vi "Drive Execute.vi"   [LabVIEW 2016]
uses:
  Drive Control Type.ctl
  Drive Notifier.ctl
  <vilib>/Rock Robotics/WPI/DriverStation/WPI_DriverStationRobotMode2.ctl
  Drive Globals.vi
  Robot Global Data.vi
types:
  T1 = typedef "WPI_MotorControlDeviceRef.ctl" = cluster{"DeviceStatus":errorcluster, "Type":T2, "PWM":cluster{"PWM Channel":T3, "DeadBand":T4}, "CAN":cluster{"Device Number":u8, "SetOutput VI Ref":variant, "GetOutput VI Ref":variant, "Enable VI Ref":variant, "Disable VI Ref":variant, "Data":variant}, "Invert":bool}
  T2 = typedef "WPI_MotorControlType.ctl" = enum16{"PWM", "CAN"}
  T3 = typedef "FPGA_DIOPWMChannel.ctl" = enum8{"PWM 0", "PWM 1", "PWM 2", "PWM 3", "PWM 4", "PWM 5", "PWM 6", "PWM 7", "PWM 8", "PWM 9", "PWM MXP 0", "PWM MXP 1", "PWM MXP 2", "PWM MXP 3", "PWM MXP 4", "PWM MXP 5", "PWM MXP 6", "PWM MXP 7", "PWM MXP 8", "PWM MXP 9", "Invalid"}
  T4 = typedef "WPI_PWMDeadband.ctl" = cluster{"Name":string, "maxPositivePwm":i32, "minPositivePwm":i32, "centerPwm":i32, "maxNegativePwm":i32, "minNegativePwm":i32, "angularRange":u16}
  T5 = typedef "Drive Control Type.ctl" = enum16{"No Op", "Fieldcentric", "Robotcentric", "Reset Wheel Position", "Reset Gyro Value", "Turn to Angle", "Drive For Time", "Drive For Time2"}
  T6 = typedef "WPI_DriverStationRobotMode2.ctl" = enum16{"Autonomous Disabled", "Autonomous Enabled", "Teleop Disabled", "Teleop Enabled", "Disconnected", "Finish", "Test Disabled", "Test Enabled", "Emergency Stopped"}
  T7 = typedef "Drive Notifier.ctl" = cluster{"Parameter 1":dbl, "Parameter 2":dbl, "Parameter 3":dbl, "Drive Control List":T5, "Parameter 4":dbl, "Gear Angle":dbl, "Parameter 6":dbl, "Parameter 7":dbl, "Parameter 8":dbl, "Parameter 9":dbl, "Robotcentric":bool, "Reset Gyro":bool, "Reset Wheels":bool, "Turn to Gear Left":bool, "Turn to Gear Center":bool, "Turn to Gear Right":bool, "Half Power":bool, "Drive Notifier":refnum<notifier>, "Step":i32}
  T8 = typedef "WPI_CANTalonSRX_GlobalStatus.ctl" = cluster{"Applied Throttle":dbl, "Module Enabled":bool, "CAN Error":errorcluster, "Closed Loop Error":dbl, "Forward Limit Switch Closed":bool, "Reverse Limit Switch Closed":bool, "Sensor Position":dbl, "Sensor Velocity":dbl, "Current":dbl, "Sticky Fault - Over Temp":bool, "Sticky Fault - Under Voltage":bool, "Sticky Fault - Forward Limit":bool, "Sticky Fault - Reverse Limit":bool, "Sticky Fault - Forward Soft Limit":bool, "Sticky Fault - Reverse Soft Limit":bool, "Brake is Enabled":bool, "Encoder Position":dbl, "Encoder Velocity":dbl, "Encoder Index Count":dbl, "Encoder A Pin State":bool, "Encoder B Pin State":bool, "Encoder Index Pin State":bool, "Analog In":dbl, "Analog In Velocity":dbl, "Temperature (C)":dbl, "Battery Voltage":dbl, "Control 5 Is Supported":bool, "Current Profile Slot Select":dbl, "Pos Div 8":bool, "Vel Div 4":bool, "Pulse Width Position":i32, "Pulse Width Velocity":i32, "Pulse Width Rise To Rise (us)":i32, "Pulse Width Rise To Fall (us)":i32, "Mot Prof Active Is Under Run":bool, "Mot Prof Active Has Under Run":bool, "Mot Prof Active Is Last":bool, "Mot Prof Active Velocity Only":bool, "Mot Prof Active Is Valid":bool, "Mot Prof Buffer Is Full":bool, "Mot Prof Active Profile Slot Select":i32, "Mot Prof NextID":i32, "Mot Prof Count":i32, "Mot Prof Active Velocity":dbl, "Mot Prof Active Position":dbl, "Mot Prof Output Enable":i32, "UsageFrame":u32, "Motion Magic Active Trajectory":cluster{"Velocity":dbl, "Position":dbl}}
  T9 = typedef "CTRE_PigeonIMU_DeviceRef.ctl" = cluster{"DeviceStatus":errorcluster, "Device Number":u8, "Type":T10, "Device ID":u32}
  T10 = typedef "CTRE_PigeonIMU_ConnectionType.ctl" = u32
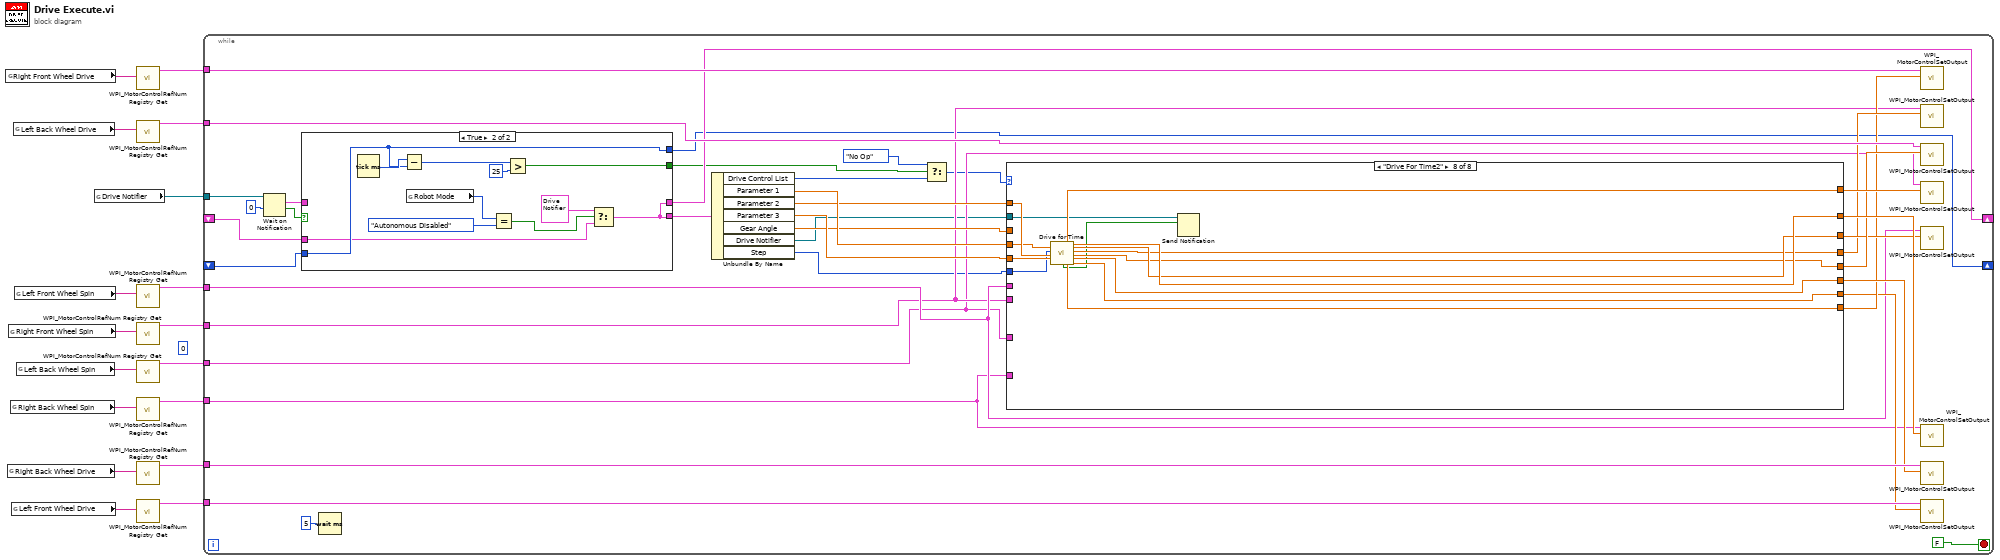
[diagram p0: block diagram]
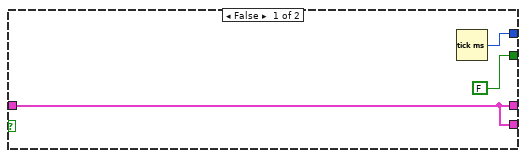
[diagram p2: hidden frame]
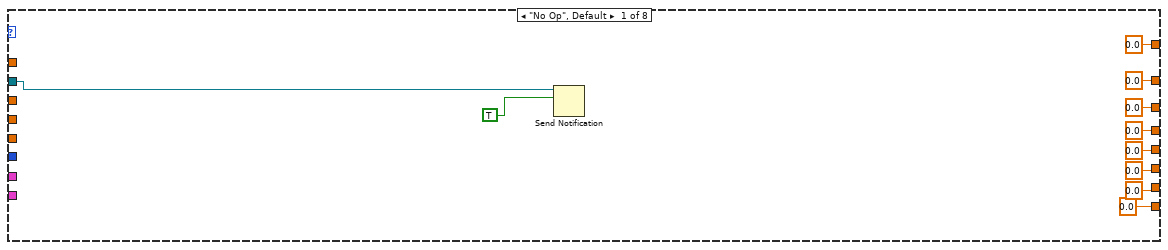
[diagram p3: hidden frame]
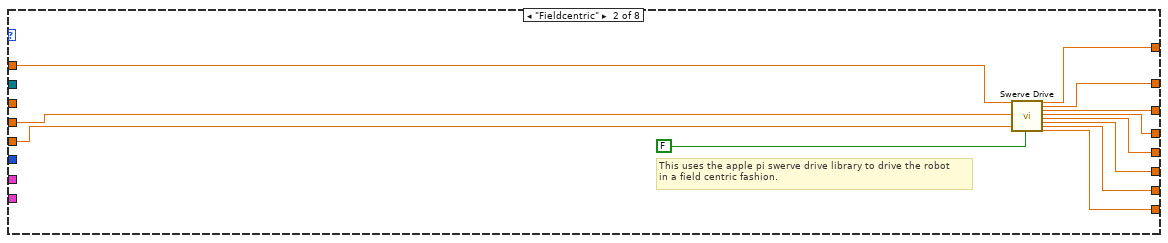
[diagram p4: hidden frame]
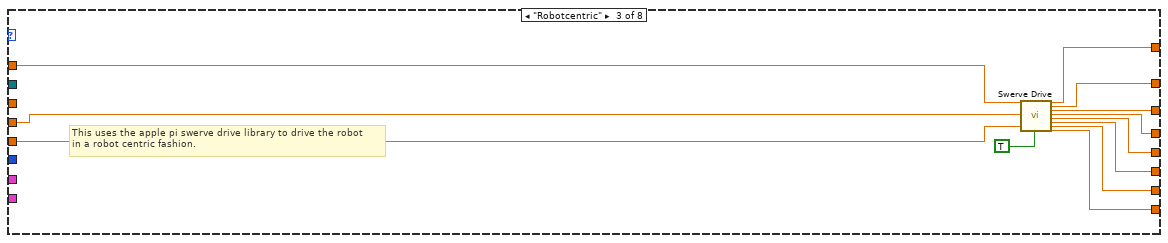
[diagram p5: hidden frame]
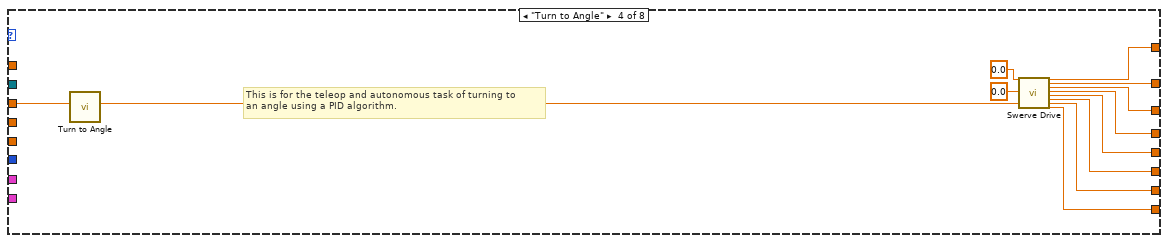
[diagram p6: hidden frame]
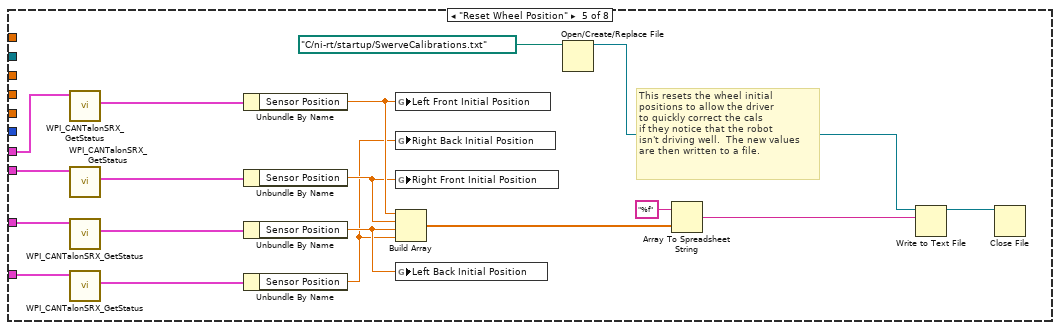
[diagram p7: hidden frame]
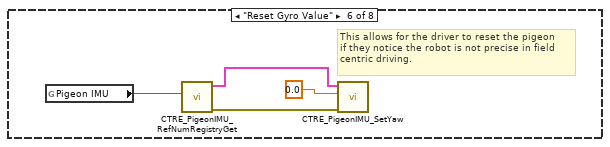
[diagram p8: hidden frame]
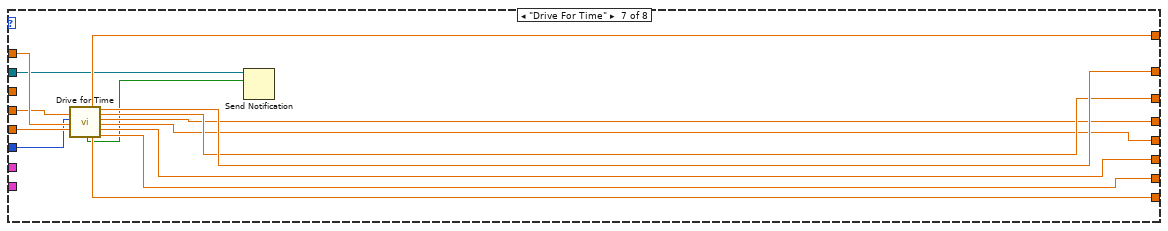
[diagram p9: hidden frame]
diagram:
  (unwired) 0
  n1 = global read "Drive Globals.vi" "Right Front Wheel Drive"() -> (w12:string)
  n2 = global read "Drive Globals.vi" "Right Back Wheel Drive"() -> (w11:string)
  n3 = global read "Drive Globals.vi" "Right Front Wheel Spin"() -> (w8:string)
  n4 = global read "Drive Globals.vi" "Right Back Wheel Spin"() -> (w6:string)
  n5 = global read "Drive Globals.vi" "Left Front Wheel Drive"() -> (w13:string)
  n6 = global read "Drive Globals.vi" "Left Back Wheel Drive"() -> (w10:string)
  n7 = global read "Drive Globals.vi" "Left Front Wheel Spin"() -> (w9:string)
  n8 = global read "Drive Globals.vi" "Left Back Wheel Spin"() -> (w7:string)
  n9 = global read "Drive Globals.vi" "Drive Notifier"() -> (w17:refnum<notifier>)
  n10 = call <vilib>:"WPI_MotorControlRefNum Registry Get.vi"("refnum name"=w12) -> ("MotorControlDevRef"=w2:T1)  [unwired: 9 in, 1 out]
  n11 = call <vilib>:"WPI_MotorControlRefNum Registry Get.vi"("refnum name"=w10) -> ("MotorControlDevRef"=w15:T1)  [unwired: 9 in, 1 out]
  n12 = call <vilib>:"WPI_MotorControlRefNum Registry Get.vi"("refnum name"=w9) -> ("MotorControlDevRef"=w1:T1)  [unwired: 9 in, 1 out]
  n13 = call <vilib>:"WPI_MotorControlRefNum Registry Get.vi"("refnum name"=w8) -> ("MotorControlDevRef"=w3:T1)  [unwired: 9 in, 1 out]
  n14 = call <vilib>:"WPI_MotorControlRefNum Registry Get.vi"("refnum name"=w7) -> ("MotorControlDevRef"=w4:T1)  [unwired: 9 in, 1 out]
  n15 = call <vilib>:"WPI_MotorControlRefNum Registry Get.vi"("refnum name"=w6) -> ("MotorControlDevRef"=w5:T1)  [unwired: 9 in, 1 out]
  n16 = call <vilib>:"WPI_MotorControlRefNum Registry Get.vi"("refnum name"=w11) -> ("MotorControlDevRef"=w14:T1)  [unwired: 9 in, 1 out]
  n17 = call <vilib>:"WPI_MotorControlRefNum Registry Get.vi"("refnum name"=w13) -> ("MotorControlDevRef"=w16:T1)  [unwired: 9 in, 1 out]
  n18 = while {
    tunnel: w17 -> [w49]
    tunnel: w16 -> [w46]
    tunnel: w15 -> [w44]
    tunnel: w14 -> [w45]
    tunnel: w5 -> [w32]
    tunnel: w4 -> [w33]
    tunnel: w3 -> [w34]
    tunnel: w2 -> [w47]
    tunnel: w1 -> [w35]
    shift-right: [w27] -> _
    shift-left: _ -> [w26]
    shift-right: [w25] -> _
    shift-left: _ -> [w24]
    stop <- FALSE stop-if-true
    n19 = Wait on Notification(notifier=w49, timeout in ms (-1)=0) -> (notification=w29:T7, timed out?=w19:bool)  [unwired: 2 in, 2 out]
    n20 = case shown="True" w19 {
      tunnel: w29 -> [w57 _]
      tunnel: [w57 w58] -> w28
      tunnel: [w57 w58] -> w27
      tunnel: w26 -> [_ w59]
      tunnel: [w56 w67] -> w25
      tunnel: w24 -> [_ w67]
      tunnel: [FALSE w64] -> w23
      frame False {
        n21 = Tick Count (ms)() -> (millisecond timer value=w56:u32)
      }
      frame True {
        n22 = Tick Count (ms)() -> (millisecond timer value=w68:u32)
        n23 = Subtract(x=w68, y=w67) -> (x-y=w66:u32)
        n24 = global read "Robot Global Data.vi" "Robot Mode"() -> (w63:T6)
        n25 = Equal?(x=w63, y=WPI_DriverStationRobotMode2."Autonomous Disabled") -> (x = y?=w61:bool)
        n26 = Greater?(x=w66, y=u32 25) -> (0:w64:bool)
        n27 = Select(t=T7 {"Parameter 1"=0.0, "Parameter 2"=0.0, "Parameter 3"=0.0, "Drive Control List"=enum."No Op", "Parameter 4"=0.0, "Gear Angle"=0.0, "Parameter 6"=0.0, "Parameter 7"=0.0, "Parameter 8"=0.0, "Parameter 9"=0.0, "Robotcentric"=FALSE, "Reset Gyro"=FALSE, "Reset Wheels"=FALSE, "Turn to Gear Left"=FALSE, "Turn to Gear Center"=FALSE, "Turn to Gear Right"=FALSE, "Half Power"=FALSE, "Drive Notifier"=refnum, "Step"=0} ("Drive Notifier"), s=w61, f=w59) -> (s? t:f=w58:T7)
      }
    }
    n28 = Wait (ms)(milliseconds to wait=u32 5) -> ()  [unwired: 1 out]
    n29 = Unbundle By Name(w28) -> ("Drive Control List"=w20:T5, "Parameter 1"=w52:dbl, "Parameter 2"=w51:dbl, "Parameter 3"=w50:dbl, "Gear Angle"=w48:dbl, "Drive Notifier"=w31:refnum<notifier>, "Step"=w18:i32)
    n30 = Select(t=Drive_Control_Type."No Op" ("f"), s=w23, f=w20) -> (s? t:f=w22:T5)
    n31 = case shown="\"Drive For Time2\"" w22 {
      tunnel: w52 -> [_ w89 w101 _ _ _ w149 w163]
      tunnel: w51 -> [_ w90 w102 _ _ _ w150 w164]
      tunnel: w50 -> [_ w88 w100 _ _ _ w148 w162]
      tunnel: w48 -> [_ _ _ w113 _ _ _ _]
      tunnel: [0.0 ("Back Left Spin Power") w87 w99 w105 _ _ w147 w161] -> w43
      tunnel: [0.0 ("Back Right Spin Power") w86 w98 w109 _ _ w146 w160] -> w42
      tunnel: [0.0 ("Back Left Motor Power") w85 w97 w108 _ _ w143 w157] -> w41
      tunnel: [0.0 ("Back Right Motor Power") w84 w96 w110 _ _ w142 w156] -> w40
      tunnel: [0.0 ("Front Left Spin Power") w83 w95 w104 _ _ w145 w159] -> w39
      tunnel: [0.0 ("Front Right Spin Power") w82 w94 w106 _ _ w144 w158] -> w38
      tunnel: [0.0 ("Front Right Motor Power") w81 w93 w107 _ _ w140 w154] -> w37
      tunnel: [0.0 ("Front Left Motor Power") w80 w92 w103 _ _ w141 w155] -> w36
      tunnel: w35 -> [_ _ _ _ w118 _ _ _]
      tunnel: w34 -> [_ _ _ _ w117 _ _ _]
      tunnel: w33 -> [_ _ _ _ w116 _ _ _]
      tunnel: w32 -> [_ _ _ _ w115 _ _ _]
      tunnel: w31 -> [w70 _ _ _ _ _ w139 w153]
      tunnel: w18 -> [_ _ _ _ _ _ w137 w151]
      frame "No Op", Default {
        n32 = Send Notification(notification=TRUE, notifier=w70) -> ()  [unwired: 1 in, 2 out]
      }
      frame "Fieldcentric" {
        # "This uses the apple pi swerve drive library to drive the robot\nin a field centric fashion."
        n33 = call "Swerve Drive.vi"("X"=w90, "Y"=w89, "Z"=w88, "Robot-Centric"=FALSE) -> ("Back Left Spin Power"=w87:dbl, "Back Right Spin Power"=w86:dbl, "Front Left Spin Power"=w83:dbl, "Front Right Spin Power"=w82:dbl, "Back Left Motor Power"=w85:dbl, "Back Right Motor Power"=w84:dbl, "Front Left Motor Power"=w80:dbl, "Front Right Motor Power"=w81:dbl)  [unwired: 16 in]
      }
      frame "Robotcentric" {
        # "This uses the apple pi swerve drive library to drive the robot\nin a robot centric fashion."
        n34 = call "Swerve Drive.vi"("X"=w102, "Y"=w101, "Z"=w100, "Robot-Centric"=TRUE) -> ("Back Left Spin Power"=w99:dbl, "Back Right Spin Power"=w98:dbl, "Front Left Spin Power"=w95:dbl, "Front Right Spin Power"=w94:dbl, "Back Left Motor Power"=w97:dbl, "Back Right Motor Power"=w96:dbl, "Front Left Motor Power"=w92:dbl, "Front Right Motor Power"=w93:dbl)  [unwired: 16 in]
      }
      frame "Turn to Angle" {
        # "This is for the teleop and autonomous task of turning to \nan angle using a PID algorithm."
        n35 = call "Turn to Angle.vi"("Target Angle"=w113) -> ("Output Rotation"=w114:dbl)  [unwired: 10 in]
        n36 = call "Swerve Drive.vi"("X"=0.0, "Y"=0.0, "Z"=w114) -> ("Back Left Spin Power"=w105:dbl, "Back Right Spin Power"=w109:dbl, "Front Left Spin Power"=w104:dbl, "Front Right Spin Power"=w106:dbl, "Back Left Motor Power"=w108:dbl, "Back Right Motor Power"=w110:dbl, "Front Left Motor Power"=w103:dbl, "Front Right Motor Power"=w107:dbl)  [unwired: 17 in]
      }
      frame "Reset Wheel Position" {
        # "This resets the wheel initial\npositions to allow the driver\nto quickly correct the cals\nif they notice that the robot\nisn't driving well.  The new values \nare then written to a file."
        n37 = call <vilib>:"WPI_CANTalonSRX_GetStatus.vi"("CAN Talon SRX Ref"=w118) -> ("Talon SRX Status"=w130:T8)  [unwired: 8 in, 2 out]
        n38 = call <vilib>:"WPI_CANTalonSRX_GetStatus.vi"("CAN Talon SRX Ref"=w117) -> ("Talon SRX Status"=w131:T8)  [unwired: 8 in, 2 out]
        n39 = call <vilib>:"WPI_CANTalonSRX_GetStatus.vi"("CAN Talon SRX Ref"=w116) -> ("Talon SRX Status"=w132:T8)  [unwired: 8 in, 2 out]
        n40 = call <vilib>:"WPI_CANTalonSRX_GetStatus.vi"("CAN Talon SRX Ref"=w115) -> ("Talon SRX Status"=w129:T8)  [unwired: 8 in, 2 out]
        n41 = Unbundle By Name(w130) -> ("Sensor Position"=w128:dbl)
        n42 = Unbundle By Name(w131) -> ("Sensor Position"=w127:dbl)
        n43 = Unbundle By Name(w132) -> ("Sensor Position"=w126:dbl)
        n44 = Unbundle By Name(w129) -> ("Sensor Position"=w125:dbl)
        n45 = global write "Drive Globals.vi" "Left Front Initial Position"(w128) -> ()
        n46 = global write "Drive Globals.vi" "Right Back Initial Position"(w125) -> ()
        n47 = global write "Drive Globals.vi" "Right Front Initial Position"(w127) -> ()
        n48 = Build Array(w128, w127, w126, w125) -> (w124:dbl[])
        n49 = global write "Drive Globals.vi" "Left Back Initial Position"(w126) -> ()
        n50 = Open/Create/Replace File(file path (use dialog)=path "C:/ni-rt/startup/SwerveCalibrations.txt" ("file (use dialog)")) -> (refnum out=w121:refnum<file>)  [unwired: 5 in, 2 out]
        n51 = Array To Spreadsheet String(array=w124, 3:"%f" ("format string")) -> (spreadsheet string=w119:string)  [unwired: 1 in]
        n52 = Write to Text File(file (use dialog)=w121, text=w119) -> (refnum out=w122:refnum<file>)  [unwired: 2 in, 2 out]
        n53 = Close File(refnum=w122) -> ()  [unwired: 1 in, 2 out]
      }
      frame "Reset Gyro Value" {
        # "This allows for the driver to reset the pigeon \nif they notice the robot is not precise in field\ncentric driving."
        n54 = global read "Drive Globals.vi" "Pigeon IMU"() -> (w133:string)
        n55 = call <vilib>:"CTRE_PigeonIMU_RefNumRegistryGet.vi"("refnum name"=w133) -> ("error out"=w134:errorcluster, "PigeonIMUDevRef"=w135:T9)  [unwired: 9 in]
        n56 = call <vilib>:"CTRE_PigeonIMU_SetYaw.vi"("error in (no error)"=w134, "Value"=0.0, "PigeonIMUDevRef"=w135) -> ()  [unwired: 7 in, 2 out]
      }
      frame "Drive For Time" {
        n57 = call "Drive for Time.vi"("Time to Run (ms)"=w149, "Step"=w137, "Drive (Throttle)"=w150, "Translation (Throttle)"=w148) -> ("Completed"=w138:bool, "Back Left Spin Power"=w147:dbl, "Front Right Motor Power"=w140:dbl, "Back Right Spin Power"=w146:dbl, "Front Left Spin Power"=w145:dbl, "Front Right Spin Power"=w144:dbl, "Back Left Motor Power"=w143:dbl, "Back Right Motor Power"=w142:dbl, "Front Left Motor Power"=w141:dbl)  [unwired: 7 in]
        n58 = Send Notification(notification=w138, notifier=w139) -> ()  [unwired: 1 in, 2 out]
      }
      frame "Drive For Time2" {
        n59 = call "Drive for Time.vi"("Time to Run (ms)"=w163, "Step"=w151, "Drive (Throttle)"=w164, "Translation (Throttle)"=w162) -> ("Completed"=w152:bool, "Back Left Spin Power"=w161:dbl, "Front Right Motor Power"=w154:dbl, "Back Right Spin Power"=w160:dbl, "Front Left Spin Power"=w159:dbl, "Front Right Spin Power"=w158:dbl, "Back Left Motor Power"=w157:dbl, "Back Right Motor Power"=w156:dbl, "Front Left Motor Power"=w155:dbl)  [unwired: 7 in]
        n60 = Send Notification(notification=w152, notifier=w153) -> ()  [unwired: 1 in, 2 out]
      }
    }
    n61 = call <vilib>:"WPI_MotorControlSetOutput.vi"("Output"=w37, "MotorControlDevRef"=w47) -> ()  [unwired: 7 in, 3 out]
    n62 = call <vilib>:"WPI_MotorControlSetOutput.vi"("Output"=w38, "MotorControlDevRef"=w34) -> ()  [unwired: 7 in, 3 out]
    n63 = call <vilib>:"WPI_MotorControlSetOutput.vi"("Output"=w41, "MotorControlDevRef"=w44) -> ()  [unwired: 7 in, 3 out]
    n64 = call <vilib>:"WPI_MotorControlSetOutput.vi"("Output"=w43, "MotorControlDevRef"=w33) -> ()  [unwired: 7 in, 3 out]
    n65 = call <vilib>:"WPI_MotorControlSetOutput.vi"("Output"=w39, "MotorControlDevRef"=w35) -> ()  [unwired: 7 in, 3 out]
    n66 = call <vilib>:"WPI_MotorControlSetOutput.vi"("Output"=w42, "MotorControlDevRef"=w32) -> ()  [unwired: 7 in, 3 out]
    n67 = call <vilib>:"WPI_MotorControlSetOutput.vi"("Output"=w40, "MotorControlDevRef"=w45) -> ()  [unwired: 7 in, 3 out]
    n68 = call <vilib>:"WPI_MotorControlSetOutput.vi"("Output"=w36, "MotorControlDevRef"=w46) -> ()  [unwired: 7 in, 3 out]
  }
